vi "GetVoltageVsCurrentGraphData.vi"(8 "error in (no error)":errorcluster, 11 "WaveformChart in":refnum<vi>) -> (0 "error out":errorcluster, 3 "Cluster":cluster{dbl[], dbl[]})   [LabVIEW 2018, in "Visualization.lvlib" / "VisualizeAcPwr.lvclass"]
uses:
  VisualizeAcPwr.lvclass
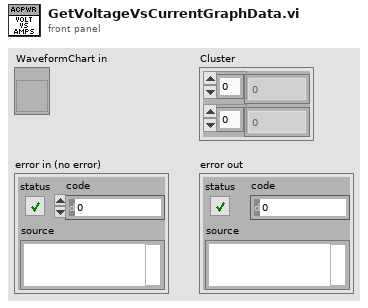
[diagram p1: front panel]
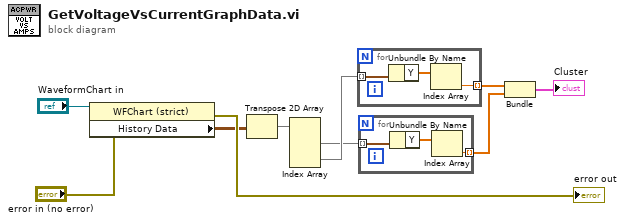
[diagram p0: block diagram]
diagram:
  n1 = property on="Property Node" class="WFChart (strict)"(reference="WaveformChart in", error in="error in (no error)") -> (error out=→"error out":errorcluster, "History Data"=w4:waveform(dbl)[][])  [unwired: 1 out]
  n2 = Transpose 2D Array(2D array=w4) -> (transposed array=w3:waveform(dbl)[][])
  n3 = Index Array(array=w3) -> (element #1=w7:waveform(dbl)[], element #2=w8:waveform(dbl)[])  [unwired: 4 in]
  n4 = for {
    tunnel: w8 -> [w13] mode=indexing
    tunnel: [w11] -> w6 mode=indexing
    n5 = Unbundle By Name(w13) -> ("Y"=w12:dbl[])
    n6 = Index Array(array=w12) -> (element=w11:dbl)  [unwired: 1 in]
  }
  n7 = for {
    tunnel: w7 -> [w16] mode=indexing
    tunnel: [w14] -> w5 mode=indexing
    n8 = Unbundle By Name(w16) -> ("Y"=w15:dbl[])
    n9 = Index Array(array=w15) -> (element=w14:dbl)  [unwired: 1 in]
  }
  n10 = Bundle(w6, w5) -> (→"Cluster":cluster{dbl[], dbl[]})  [unwired: 1 in]
